vi "Actor Core.vi"(8 "error in":errorcluster, 11 "Nested in":refnum<class "CAFE_MEX_ESP.lvclass">) -> (0 "error out":errorcluster, 3 "Actor out":refnum<class "Actor.lvclass">)   [LabVIEW 2019, in "CAFE_MEX_ESP.lvlib" / "CAFE_MEX_ESP.lvclass"]
doc: "(<B>Filename</B>: Actor Framework.lvlib:Actor.lvclass:Actor Core.vi)\n\nReceives messages to the actor, reacts to them, and initiates any error handling that may shut the actor down.\n\nDescendant classes may override this VI to append parallel tasks for the actor to complete while it handles messages. Overrides use the Call Parent Method node."
uses:
  CAFE_MEX_ESP.lvclass
  C:/Program Files (x86)/National Instruments/LabVIEW 2019/vi.lib/ActorFramework/Actor/Actor.lvclass
  <vilib>/ActorFramework/Actor/Actor.lvclass
  DATABASE/DATABASE/DATABASE.lvclass
  CAFE_MEX_ESP.lvclass/CAFE_MEX_ESP.ctl
  <vilib>/ActorFramework/Actor/Actor.lvclass/Actor.ctl
  <vilib>/ActorFramework/Message Enqueuer/Message Enqueuer.lvclass/Message Enqueuer.ctl
  CAFE_MEX_ESP Messages/MANDAR_DIRECCION Msg/MANDAR_DIRECCION Msg.lvclass/MANDAR_DIRECCION Msg.ctl
  <vilib>/ActorFramework/Message Enqueuer/Init from Existing Queue.vi
  <vilib>/ActorFramework/Message Enqueuer/Enqueue.vi
  <vilib>/ActorFramework/Stop Msg/Stop Msg.lvclass
  C:/Program Files (x86)/National Instruments/LabVIEW 2019/vi.lib/ActorFramework/Message/Message.lvclass
  CAFE_MEX_ESP Messages/MANDAR_DIRECCION Msg/MANDAR_DIRECCION Msg.lvclass
  <vilib>/ActorFramework/Message Priority Queue/Priority Enqueue.vi
  <vilib>/ActorFramework/Message Enqueuer/Message Enqueuer.lvclass
panel:
  out "MERCANCIA":string[][](array[string])
  in  "SOLICITAR MERCANCIA":bool
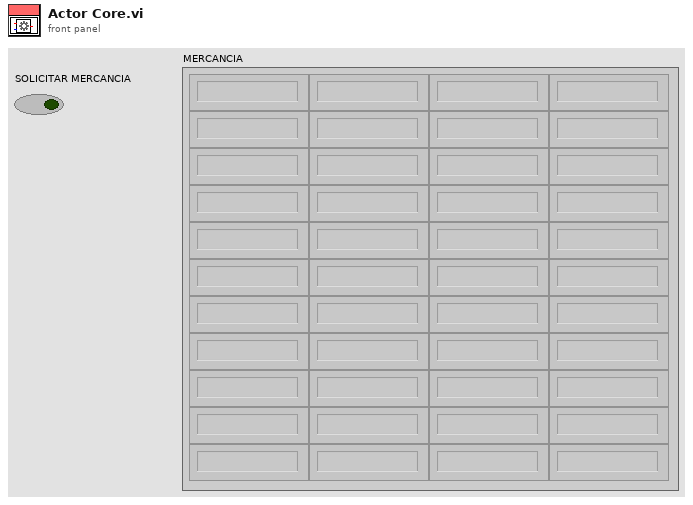
[diagram p1: front panel]
types:
  T1 = cluster{"Stop":refnum<user-event>, "MERCANCIA":refnum<user-event>}
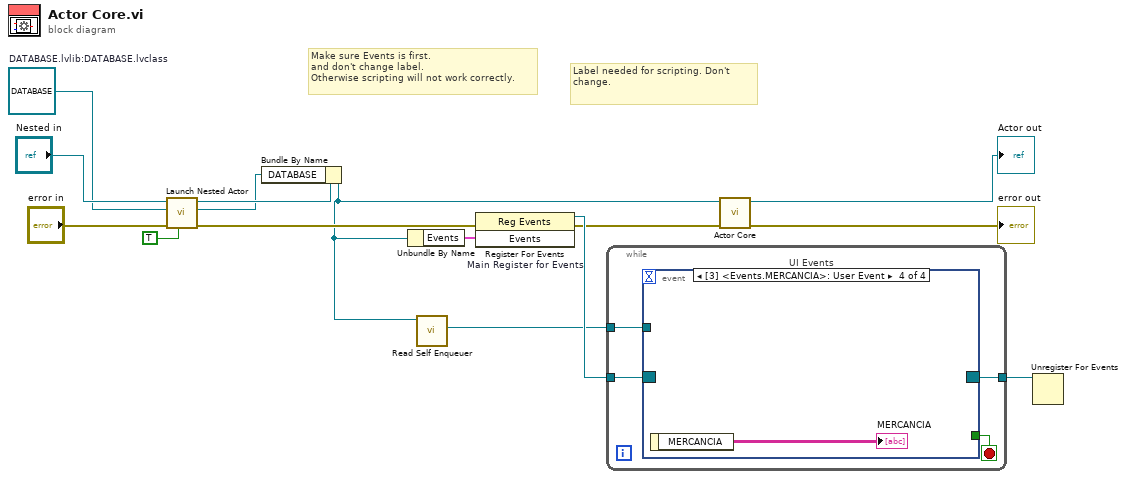
[diagram p0: block diagram]
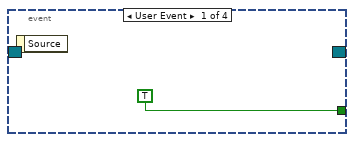
[diagram p2: hidden frame]
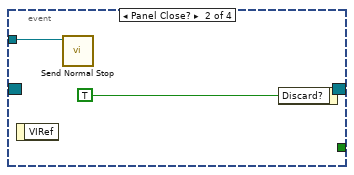
[diagram p3: hidden frame]
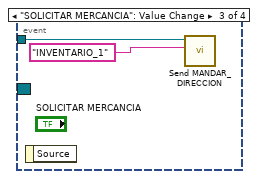
[diagram p4: hidden frame]
diagram:
  w4 = refnum<class "DATABASE.lvclass"> refnum  # DATABASE.lvlib:DATABASE.lvclass
  # "Label needed for scripting. Don't change."
  # "Make sure Events is first.\nand don't change label.\nOtherwise scripting will not work correctly."
  n1 = call <vilib>:"Launch Nested Actor.vi"("Open Actor Core front panel? (F)"=TRUE, "error in (no error)"="error in", "Nested Actor"=w4, "Caller Actor in"="Nested in") -> ("error out"=w7:errorcluster, "Nested Actor's Enqueuer"=w2:refnum<class "Message Enqueuer.lvclass">, "Caller Actor out"=w5:refnum<class "CAFE_MEX_ESP.lvclass">)  [unwired: 5 in]
  n2 = Bundle By Name(cluster=w5, "DATABASE"=w2) -> (w3:refnum<class "CAFE_MEX_ESP.lvclass">)
  n3 = Unbundle By Name(w3) -> ("Events"=w12:T1)
  n4 = call <vilib>:"Read Self Enqueuer.vi"("Actor"=w3) -> ("Self Enqueuer"=w10:refnum<class "Message Enqueuer.lvclass">)  [unwired: 10 in]
  n5 = register-events "Main Register for Events"(error in=w7, w12) -> (reference out=w13:refnum<event-registration>, error out=w8:errorcluster)  [unwired: 1 in]
  n6 = while {
    tunnel: w13 -> [w19]
    tunnel: [w17] -> w11
    tunnel: w10 -> [w16]
    stop <- w18 stop-if-true
    n7 = event "UI Events" shown="[3] <Events.MERCANCIA>: User Event" {
      selector: w19 -> [_ _ _ _]
      dyn-events: [_ _ _ _] -> w17
      timeout: _ -> [_ _ _ _]
      tunnel: [TRUE _ _ _] -> w18
      tunnel: w16 -> [_ w21 w24 _]
      event User Event {
        n8 = event-data() -> ()  [unwired: 1 in, 1 out]
      }
      event Panel Close? {
        n9 = event-data() -> ()  [unwired: 1 in, 1 out]
        n10 = call <vilib>:"Send Normal Stop.vi"("Message Enqueuer"=w21) -> ()  [unwired: 10 in, 1 out]
        n11 = event-data("Discard?"=TRUE) -> ()  [unwired: 1 in, 1 out]
      }
      event "SOLICITAR MERCANCIA": Value Change {
        n12 = event-data() -> ()  [unwired: 1 in, 1 out]
        n13 = call "Send MANDAR_DIRECCION.vi"("BASE_DE_DATOS"="INVENTARIO_1", "Message Enqueuer"=w24) -> ()  [unwired: 8 in, 2 out]
      }
      event User Event {
        n14 = event-data() -> ("MERCANCIA"=→"MERCANCIA":string[][])  [unwired: 1 in]
      }
    }
  }
  n15 = call-parent "Actor Core.vi"("error in"=w8, "Actor in"=w3) -> ("error out"=→"error out":errorcluster, "Actor out"=→"Actor out":refnum<class "Actor.lvclass">)  [unwired: 8 in]
  n16 = Unregister For Events(event registration refnum=w11) -> ()  [unwired: 1 in, 1 out]
